vi "Init Modules.vi"(8 "error in (no error)":errorcluster, 9 "Message Queues in":T16, 11 "Settings":T1={"Support"={"Save Configuration"={"Log File Base Path"=path "", "TDMS File Reference"=refnum, "Reset"=FALSE, "Wait"=0.0, "Start Time"=0.0, "Update Rate"=1, "Channel Names"=[], "System Preset"=variant}, "LOG Configuration"={"LOG REF"=refnum, "Writer Queue"=refnum, "Log Path"=path "", "LOG"=FALSE}, "ALARM Configuration"={"LOG REF"=refnum, "Writer Queue"=refnum, "Log Path"=path "", "UPS standby"=FALSE, "status code"=5001, "SP"=[], "Over Sens Status"=[]}, "User Details"=[], "Radome Type"="", "Timer Configuration"={"Wait"=0.0, "Next Step"="", "Writer Queue"=refnum, "Reset"=FALSE, "VISA resource"="", "Status"=[], "Valve Time"=[], "Timer queue"=refnum, "Current valve"=0, "Enable"=FALSE}}, "Process"={"Test Configuration"={"current Step"=0, "Wait"=0.0, "Next Step"="", "Writer Queue"=refnum, "Reset"=FALSE, "SEQ Time"=0, "General Reset"=FALSE, "Cycles"=0, "Status"=[], "Ready"=[], "Backward"=FALSE, "Current SP"=[], "System Preset"={"Test Configuration"={"Cycles"=0, "Z Up"=0.0, "SP List"=[], "Operator"="", "Point Delay"=0, "Z Up 2"=0.0, "Cleaning In"=0.0, "Cleaning Out"=0.0, "Cleaning Cycles"=0}, "Test_Start_date"=""}, "Test Type"=enum."Calibration", "Sample Count"=0, "Local Queues"={"Cycles queue"=refnum, "Step queue"=refnum, "RES Queue"=refnum, "Clean queue"=refnum, "PS Scan queue"=refnum}, "current Clean"=0, "PS Measure Plan"=[]}}, "Report Configuration"={"Test Setting"={"Test_Num"=0, "Test_ID"=0, "Proc_ID"=0, "Max Force"=0.0, "User"="", "SN"="", "Date"=""}, "Measurements"=[], "LOG REF"=refnum, "Report Template"=path "", "Save Report path"=path "", "Data File Path"=path "", "Popup Dialog"=FALSE}, "History Data"={"Tests"=[], "Test Name"=""}, "Motor Configuration"={"Tango HW"={"VISA resource"="", "Baud Rate (115200)"=2, "lAnInterfaceType"=0, "bAShowProt"=15}, "Writer Queue"=refnum, "Status"=FALSE, "Abs Position"=[], "Axis Velocity"={"dX"=0.0, "dY"=0.0, "dZ"=0.0, "dA"=0.0}, "acceleration "=0.0, "Z direction"=enum."Up", "Position Mode"="", "plLSID"=0}, "PalmSense  Configuration"={"PalmSens.lvclass"=refnum, "Writer Queue"=refnum, "Enable"=FALSE, "Is Measuring Ref"=refnum, "Method"={"Name"="", "Method Ref"=variant}, "PS Live Curve Result"=refnum}, "Hiden Scanner Resources"={"Link"={"Connection"=enum."USB", "Host or IP address (TCP/IP)"="", "Port (Serial/USB)"="COM1"}, "VISA resource"="", "Writer Queue"=refnum, "Status"=FALSE}, "MFC Configuration"={"MFC Definition"={"MFC Port"="", "MFC Enable"=TRUE, "Baud Rate"=0, "Interface type"=enum."RS-485", "Address"=0}, "Set Point Options"={"Setpoint Value"=0.0, "Mass Flow EU 2"="", "Setpoint Source"="", "Valve Mode"=""}, "Writer Queue"=refnum, "Enable"=FALSE, "Update Rate"=0, "MRC Chamber Enable"=FALSE, "Selected Gas"="", "Address String"=""}, "Pump Configuration"={"Pump  name"=[], "Writer Queue"=refnum, "Pump Info"={"Pump Type"="", "Speed"=0, "Direction"=0, "Running"=FALSE}, "Current Pump Name"="", "Wait"=0.0, "Next Step"="", "Reset"=FALSE}} {"Pump Configuration"."Pump Info"."Direction" items=["CW", "CCW"]; "Pump Configuration"."Pump Info"."Speed" format="%03.0f"; "MFC Configuration"."Set Point Options"."Setpoint Value" min=0.0 max=0.62495 format="%.5f"; "Process"."Test Configuration"."PS Measure Plan" items=["Pretreatment settings (PS)", "Linear Sweep Voltammetry (LSV)", "Differential Pulse Voltammetry (DPV)", "Cyclic Voltammetry (CV)", "Chronoamperometry (CA)", "Chronopotentiometry (CP)", "El Imp Spectroscopy (EIS)"]; "Process"."Test Configuration"."System Preset"."Test Configuration"."SP List" format="%#.1g"; "Support"."Save Configuration"."Update Rate" min=1 max=10 step=1}) -> (0 "error out":errorcluster)   [LabVIEW 2020]
uses:
  Message Queue/All Message Queues.ctl
  Message Queue/Message Cluster.ctl
  Settings/Settings.ctl
  <instrlib>/PalmSens SDK for LabVIEW 5.10/PalmSens/PalmSens.lvclass
  Logging/Save Configuration.ctl
  LOG/LOG Configuration.ctl
  ALARM/ALARM Configuration.ctl
  Valve Control/AM Configuration.ctl
  Test Driver/Test Driver Configuration.ctl
  Test Driver/System Preset.ctl
  Test Driver/Test Type.ctl
  Report/REP Configuration.ctl
  Report/Test Setting.ctl
  MOTOR/PS Hardware Configuration.ctl
  DMM/PalmSense Hardware Configuration.ctl
  Hiden Scanner/Scanner Hardware Configuration.ctl
  MRC/MRC Configuration.ctl
  WM Pump/Pump Hardware Configuration.ctl
  REF Single  Name to ref convert.vi
  Message Queue/Enqueue Message (Single).vi
  Message Queue/Message Queue.lvlib
  Settings/Settings.lvlib
  Logging/SAVE.lvlib
  LOG/LOG.lvlib
  ALARM/QCT ALARM.lvlib
  Report/Report.lvlib
  MOTOR/MOTOR.lvlib
  Test Driver/Test Driver.lvlib
  DMM/PalmSens.lvlib
  Hiden Scanner/Hiden Scanner.lvlib
  Valve Control/Valve Control.lvlib
  MRC/MRC Module.lvlib
  WM Pump/Pump.lvlib
panel:
  in  "CMDs":string(combo)="ALARM"
  # "X"
  # "Y"
  # "Cycles"
  # "Point Delay"
  # "Up"
  # "Down"
  # "Z Axes"
  # "#C"
  # "In"
  # "Out"
  # "Cleaning [sec]"
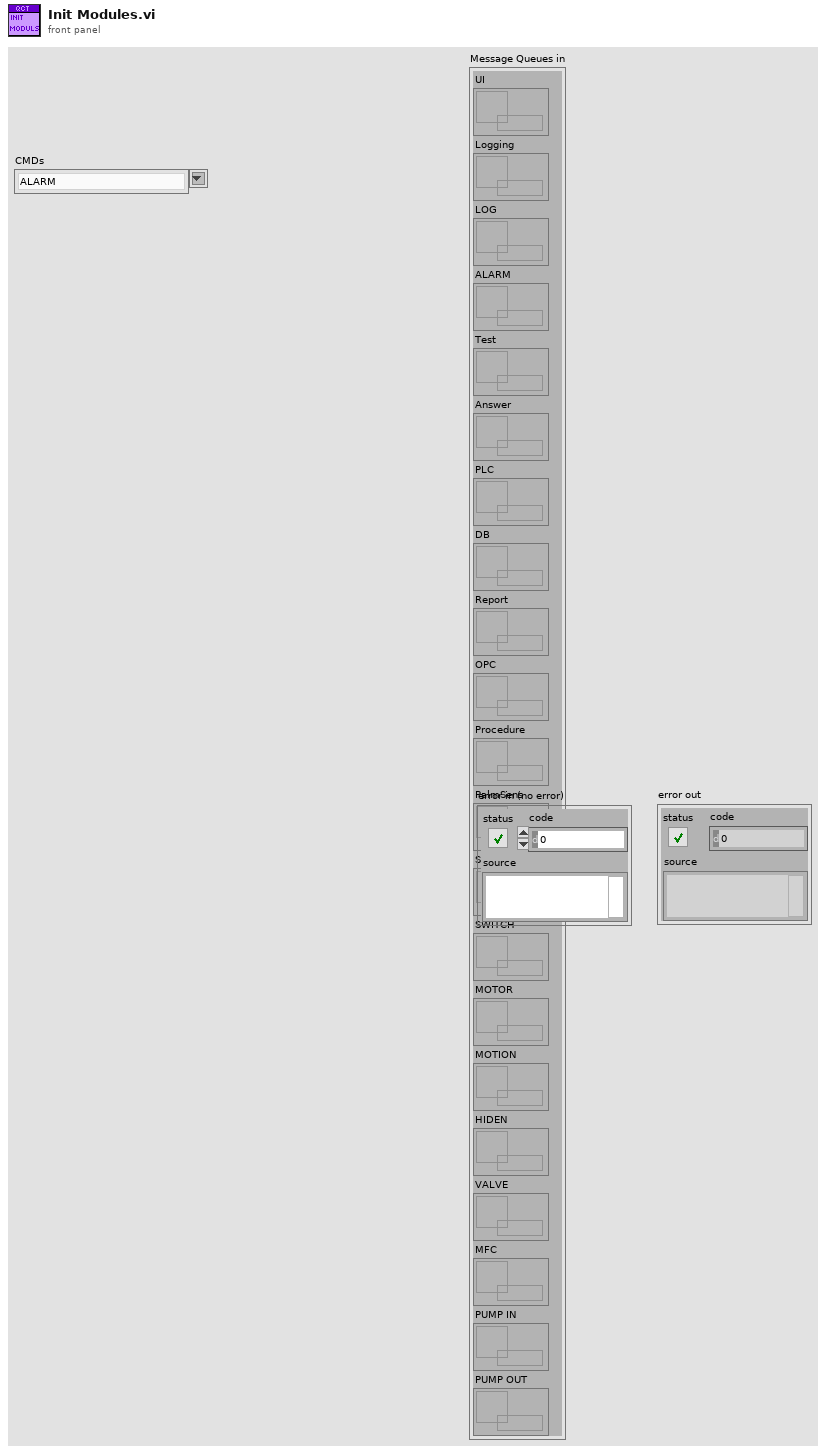
[diagram p1: front panel]
types:
  T1 = typedef "Settings.lvlib/Settings.ctl" = cluster{"Support":cluster{"Save Configuration":T2, "LOG Configuration":T3, "ALARM Configuration":T4, "User Details":string[], "Radome Type":string, "Timer Configuration":T5}, "Process":cluster{"Test Configuration":T6}, "Report Configuration":T9, "History Data":cluster{"Tests":string[][], "Test Name":string}, "Motor Configuration":T11, "PalmSense  Configuration":T12, "Hiden Scanner Resources":T13, "MFC Configuration":T14, "Pump Configuration":T15}
  T2 = typedef "SAVE.lvlib/Save Configuration.ctl" = cluster{"Log File Base Path":path, "TDMS File Reference":refnum<k34>, "Reset":bool, "Wait":dbl, "Start Time":dbl, "Update Rate":u16, "Channel Names":string[], "System Preset":variant}
  T3 = typedef "LOG.lvlib/LOG Configuration.ctl" = cluster{"LOG REF":refnum<vi>, "Writer Queue":refnum<queue>, "Log Path":path, "LOG":bool}
  T4 = typedef "QCT ALARM.lvlib/ALARM Configuration.ctl" = cluster{"LOG REF":refnum<vi>, "Writer Queue":refnum<queue>, "Log Path":path, "UPS standby":bool, "status code":i32, "SP":dbl[], "Over Sens Status":dbl[]}
  T5 = typedef "Valve Control.lvlib/AM Configuration.ctl" = cluster{"Wait":dbl, "Next Step":string, "Writer Queue":refnum<queue>, "Reset":bool, "VISA resource":refnum<visa-resource-name>, "Status":bool[], "Valve Time":dbl[], "Timer queue":refnum<queue>, "Current valve":i32, "Enable":bool}
  T6 = typedef "Test Driver.lvlib/Test Driver Configuration.ctl" = cluster{"current Step":i32, "Wait":dbl, "Next Step":string, "Writer Queue":refnum<queue>, "Reset":bool, "SEQ Time":i32, "General Reset":bool, "Cycles":i32, "Status":bool[], "Ready":bool[], "Backward":bool, "Current SP":dbl[], "System Preset":T7, "Test Type":T8, "Sample Count":i32, "Local Queues":cluster{"Cycles queue":refnum<queue>, "Step queue":refnum<queue>, "RES Queue":refnum<queue>, "Clean queue":refnum<queue>, "PS Scan queue":refnum<queue>}, "current Clean":i32, "PS Measure Plan":u16[]}
  T7 = typedef "System Preset.ctl" = cluster{"Test Configuration":cluster{"Cycles":i32, "Z Up":dbl, "SP List":dbl[][], "Operator":string, "Point Delay":i32, "Z Up 2":dbl, "Cleaning In":dbl, "Cleaning Out":dbl, "Cleaning Cycles":i32}, "Test_Start_date":string}
  T8 = typedef "Test Driver.lvlib/Test Type.ctl" = enum16{"Calibration", "Test"}
  T9 = typedef "Report.lvlib/REP Configuration.ctl" = cluster{"Test Setting":T10, "Measurements":string[][], "LOG REF":refnum<vi>, "Report Template":path, "Save Report path":path, "Data File Path":path, "Popup Dialog":bool}
  T10 = typedef "Report.lvlib/Test Setting.ctl" = cluster{"Test_Num":i32, "Test_ID":i32, "Proc_ID":i32, "Max Force":dbl, "User":string, "SN":string, "Date":string}
  T11 = typedef "MOTOR.lvlib/PS Hardware Configuration.ctl" = cluster{"Tango HW":cluster{"VISA resource":refnum<visa-resource-name>, "Baud Rate (115200)":i32, "lAnInterfaceType":i32, "bAShowProt":i32}, "Writer Queue":refnum<queue>, "Status":bool, "Abs Position":i32[], "Axis Velocity":cluster{"dX":dbl, "dY":dbl, "dZ":dbl, "dA":dbl}, "acceleration ":dbl, "Z direction":enum16{"Up", "Down"}, "Position Mode":string, "plLSID":i32}
  T12 = typedef "PalmSens.lvlib/PalmSense Hardware Configuration.ctl" = cluster{"PalmSens.lvclass":refnum<class "PalmSens.lvclass">, "Writer Queue":refnum<queue>, "Enable":bool, "Is Measuring Ref":refnum<vi>, "Method":cluster{"Name":string, "Method Ref":variant}, "PS Live Curve Result":refnum<vi>}
  T13 = typedef "Hiden Scanner.lvlib/Scanner Hardware Configuration.ctl" = cluster{"Link":cluster{"Connection":enum16{"Serial", "TCP/IP", "USB"}, "Host or IP address (TCP/IP)":string, "Port (Serial/USB)":string}, "VISA resource":refnum<visa-resource-name>, "Writer Queue":refnum<queue>, "Status":bool}
  T14 = typedef "MRC Module.lvlib/MRC Configuration.ctl" = cluster{"MFC Definition":cluster{"MFC Port":refnum<visa-resource-name>, "MFC Enable":bool, "Baud Rate":i32, "Interface type":enum32{"RS-485", "RS-232"}, "Address":i32}, "Set Point Options":cluster{"Setpoint Value":dbl, "Mass Flow EU 2":string, "Setpoint Source":string, "Valve Mode":string}, "Writer Queue":refnum<queue>, "Enable":bool, "Update Rate":u32, "MRC Chamber Enable":bool, "Selected Gas":string, "Address String":string}
  T15 = typedef "Pump.lvlib/Pump Hardware Configuration.ctl" = cluster{"Pump  name":refnum<visa-resource-name>[], "Writer Queue":refnum<queue>, "Pump Info":cluster{"Pump Type":string, "Speed":i32, "Direction":u16, "Running":bool}, "Current Pump Name":refnum<visa-resource-name>, "Wait":dbl, "Next Step":string, "Reset":bool}
  T16 = typedef "Message Queue.lvlib/All Message Queues.ctl" = cluster{"UI":refnum<queue>, "Logging":refnum<queue>, "LOG":refnum<queue>, "ALARM":refnum<queue>, "Test":refnum<queue>, "Answer":refnum<queue>, "PLC":refnum<queue>, "DB":refnum<queue>, "Report":refnum<queue>, "OPC":refnum<queue>, "Procedure":refnum<queue>, "PalmSens":refnum<queue>, "SYS 7000 Reader":refnum<queue>, "SWITCH":refnum<queue>, "MOTOR":refnum<queue>, "MOTION":refnum<queue>, "HIDEN":refnum<queue>, "VALVE":refnum<queue>, "MFC":refnum<queue>, "PUMP IN":refnum<queue>, "PUMP OUT":refnum<queue>}
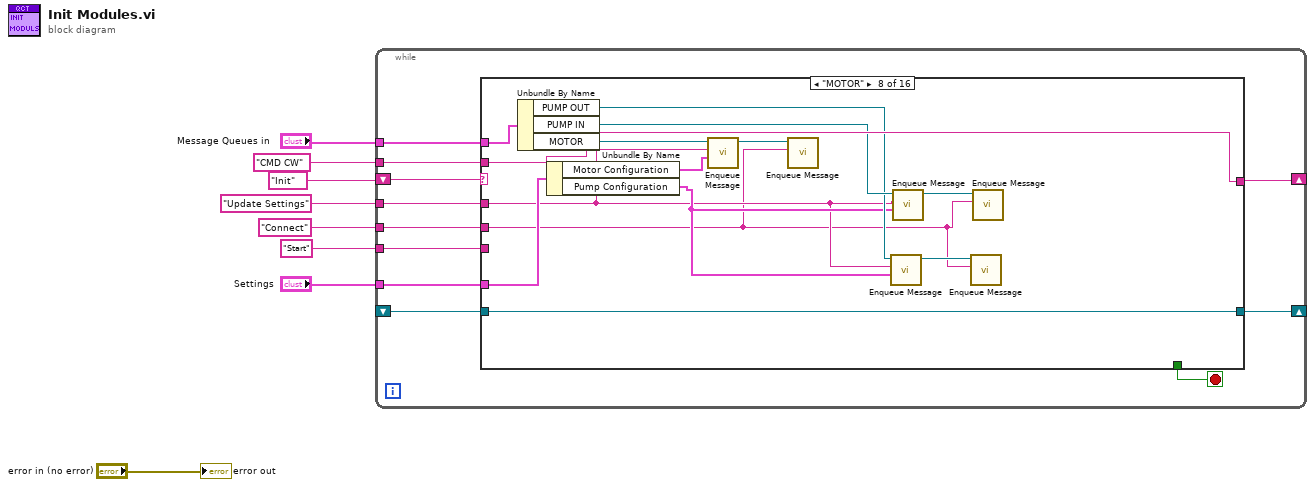
[diagram p0: block diagram]
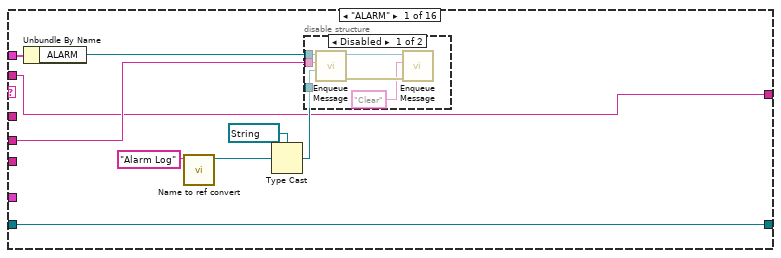
[diagram p2: hidden frame]
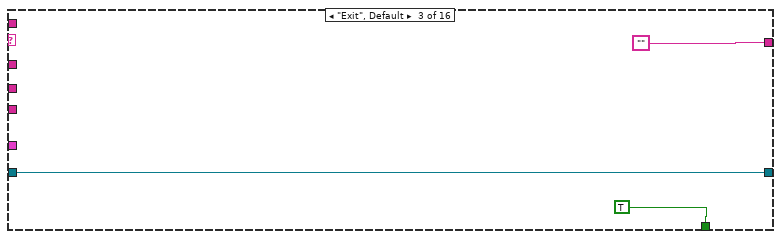
[diagram p5: hidden frame]
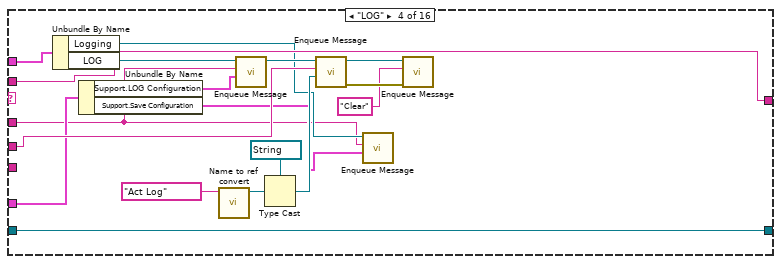
[diagram p6: hidden frame]
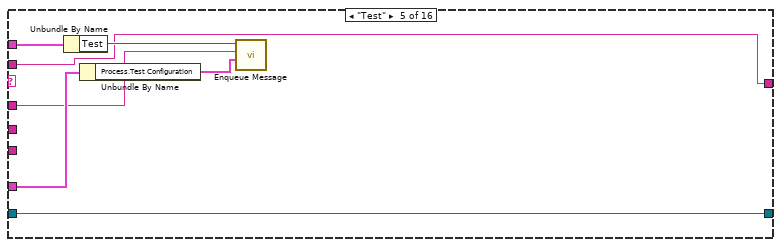
[diagram p7: hidden frame]
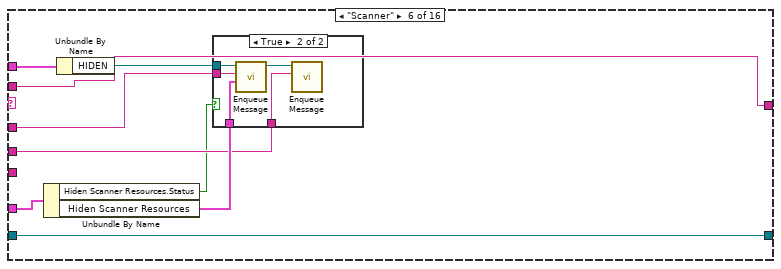
[diagram p8: hidden frame]
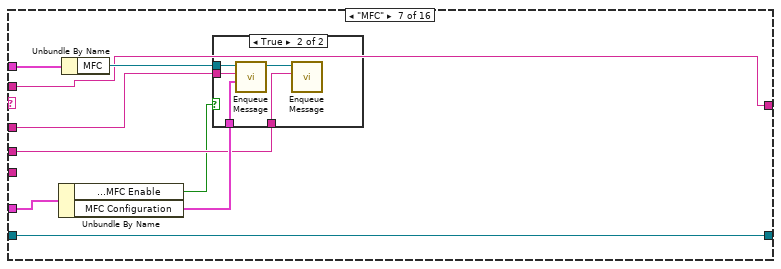
[diagram p10: hidden frame]
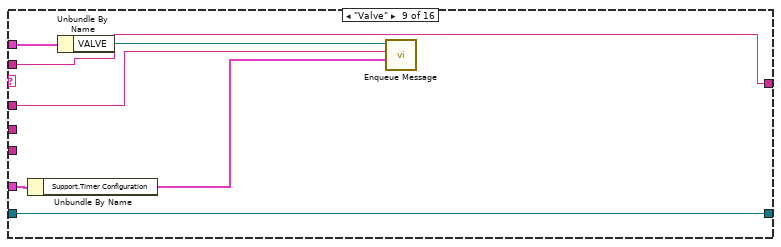
[diagram p12: hidden frame]
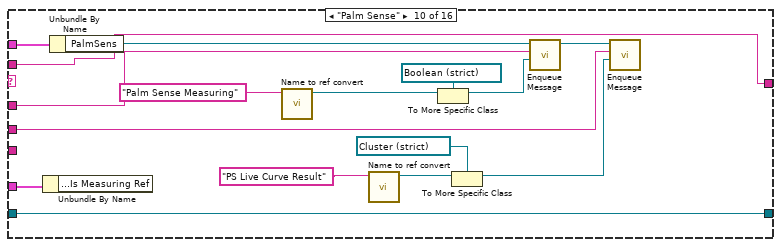
[diagram p13: hidden frame]
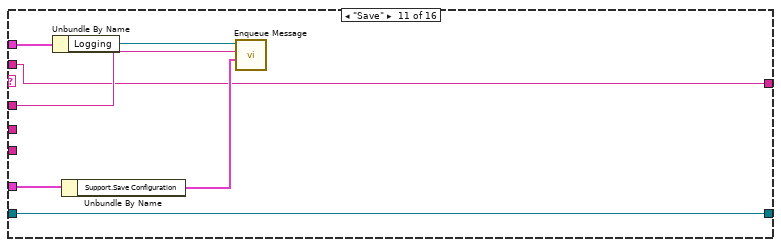
[diagram p14: hidden frame]
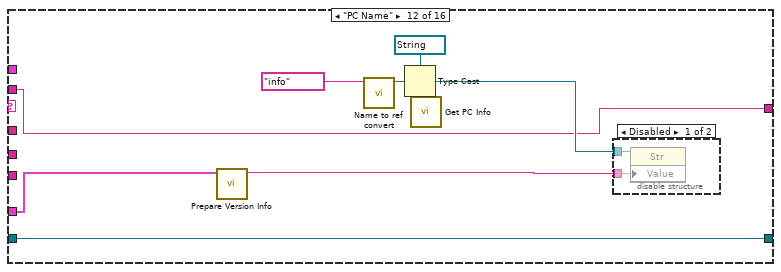
[diagram p15: hidden frame]
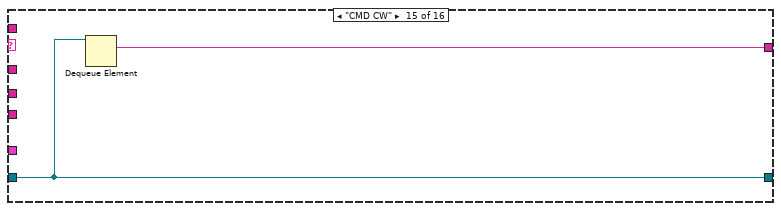
[diagram p19: hidden frame]
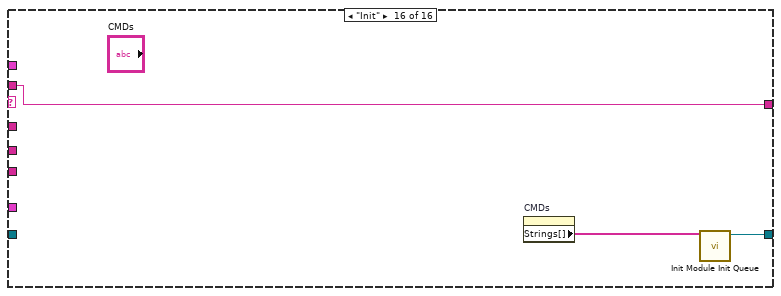
[diagram p20: hidden frame]
diagram:
  n1 = while {
    tunnel: "Message Queues in" -> [w18]
    tunnel: "Update Settings" ("Message") -> [w17]
    tunnel: "Settings" -> [w16]
    tunnel: "Connect" ("Message") -> [w15]
    shift-right: [w9] -> _
    shift-left: "Init" ("Combo Box") -> [w19]
    tunnel: "Start" ("Message") -> [w13]
    shift-right: [w11] -> _
    shift-left: _ -> [w12]
    tunnel: "CMD CW" ("Message") -> [w10]
    stop <- w14 stop-if-true
    n2 = case shown="\"MOTOR\"" w19 {
      tunnel: w18 -> [w28 _ _ w57 w64 w73 w87 w106 w113 w129 w136 _ _ _ _ _]
      tunnel: w17 -> [_ _ _ w40 w61 w70 w84 w94 w110 w125 w133 _ _ _ _ _]
      tunnel: w16 -> [_ _ _ w51 w63 w72 w86 w105 w112 w128 w135 w138 _ _ _ _]
      tunnel: w15 -> [w24 _ _ w52 _ w66 w80 w93 _ w122 _ _ _ _ _ _]
      tunnel: [w20 w35 "" w44 w58 w67 w81 w100 w107 w123 w130 w139 w147 w149 w151 w153] -> w9
      tunnel: [_ _ TRUE _ _ _ _ _ _ _ _ _ _ _ _ _] -> w14
      tunnel: w13 -> [_ _ _ _ _ _ _ _ _ _ _ _ _ _ _ _]
      tunnel: [w21 w36 w37 w45 w59 w68 w82 w101 w108 w124 w131 w140 w148 w150 w152 w154] -> w11
      tunnel: w12 -> [w21 w36 w37 w45 w59 w68 w82 w101 w108 w124 w131 w140 w148 w150 w152 _]
      tunnel: w10 -> [w20 w35 _ w44 w58 w67 w81 w100 w107 w123 w130 w139 w147 w149 _ w153]
      frame "ALARM" {
        n3 = Unbundle By Name(w28) -> ("ALARM"=w27:refnum<queue>)
        n4 = call-poly "Name to ref convert.vi"("name"="Alarm Log") -> ("First REF"=w22:refnum<vi>)  [unwired: 10 in]
        n5 = Type Cast(type=refnum<vi> refnum ("LOG"), x=w22) -> (*(type *) &x=w25:refnum<vi>)
        n6 = disable-structure shown="Disabled" {
          disable-tunnel: w27 -> [w34 _]
          disable-tunnel: w25 -> [w33 _]
          disable-tunnel: w24 -> [w29 _]
          frame Disabled {
            n7 = call-poly "Enqueue Message.vi"("Message Data"=w33, "Message"=w29, "Message Queue"=w34) -> ("error out"=w31:errorcluster, "dup Message Queue"=w32:refnum<queue>)  [unwired: 7 in]
            n8 = call-poly "Enqueue Message.vi"("error in (no error)"=w31, "Message"="Clear" ("Ready..."), "Message Queue"=w32) -> ()  [unwired: 7 in, 2 out]
          }
          frame Enabled {
          }
        }
      }
      frame "Activation" {
      }
      frame "Exit", Default {
      }
      frame "LOG" {
        n9 = Unbundle By Name(w57) -> ("Logging"=w42:refnum<queue>, "LOG"=w50:refnum<queue>)
        n10 = Unbundle By Name(w51) -> ("Support.LOG Configuration"=w48:T3, "Support.Save Configuration"=w41:T2)
        n11 = call-poly "Name to ref convert.vi"("name"="Act Log") -> ("First REF"=w46:refnum<vi>)  [unwired: 10 in]
        n12 = call-poly "Enqueue Message.vi"("Message Data"=w48, "Message"=w40, "Message Queue"=w50) -> ("dup Message Queue"=w49:refnum<queue>)  [unwired: 7 in, 1 out]
        n13 = Type Cast(type=refnum<vi> refnum ("LOG"), x=w46) -> (*(type *) &x=w55:refnum<vi>)
        n14 = call-poly "Enqueue Message.vi"("Message Data"=w55, "Message"=w52, "Message Queue"=w49) -> ("error out"=w53:errorcluster, "dup Message Queue"=w54:refnum<queue>)  [unwired: 7 in]
        n15 = call-poly "Enqueue Message.vi"("Message Data"=w41, "Message"=w40, "Message Queue"=w42) -> ()  [unwired: 7 in, 2 out]
        n16 = call-poly "Enqueue Message.vi"("error in (no error)"=w53, "Message"="Clear" ("Ready..."), "Message Queue"=w54) -> ()  [unwired: 7 in, 2 out]
      }
      frame "Test" {
        n17 = Unbundle By Name(w64) -> ("Test"=w62:refnum<queue>)
        n18 = Unbundle By Name(w63) -> ("Process.Test Configuration"=w60:T6)
        n19 = call-poly "Enqueue Message.vi"("Message Data"=w60, "Message"=w61, "Message Queue"=w62) -> ()  [unwired: 7 in, 2 out]
      }
      frame "Scanner" {
        n20 = Unbundle By Name(w72) -> ("Hiden Scanner Resources.Status"=w65:bool, "Hiden Scanner Resources"=w69:T13)
        n21 = Unbundle By Name(w73) -> ("HIDEN"=w71:refnum<queue>)
        n22 = case shown="True" w65 {
          tunnel: w71 -> [_ w78]
          tunnel: w70 -> [_ w77]
          tunnel: w69 -> [_ w76]
          tunnel: w66 -> [_ w74]
          frame False {
          }
          frame True {
            n23 = call-poly "Enqueue Message.vi"("Message Data"=w76, "Message"=w77, "Message Queue"=w78) -> ("dup Message Queue"=w75:refnum<queue>)  [unwired: 7 in, 1 out]
            n24 = call-poly "Enqueue Message.vi"("Message"=w74, "Message Queue"=w75) -> ()  [unwired: 8 in, 2 out]
          }
        }
      }
      frame "MFC" {
        n25 = Unbundle By Name(w86) -> ("MFC Configuration.MFC Definition.MFC Enable"=w79:bool, "MFC Configuration"=w83:T14)
        n26 = Unbundle By Name(w87) -> ("MFC"=w85:refnum<queue>)
        n27 = case shown="True" w79 {
          tunnel: w85 -> [_ w92]
          tunnel: w84 -> [_ w91]
          tunnel: w83 -> [_ w90]
          tunnel: w80 -> [_ w88]
          frame False {
          }
          frame True {
            n28 = call-poly "Enqueue Message.vi"("Message Data"=w90, "Message"=w91, "Message Queue"=w92) -> ("dup Message Queue"=w89:refnum<queue>)  [unwired: 7 in, 1 out]
            n29 = call-poly "Enqueue Message.vi"("Message"=w88, "Message Queue"=w89) -> ()  [unwired: 8 in, 2 out]
          }
        }
      }
      frame "MOTOR" {
        n30 = Unbundle By Name(w106) -> ("PUMP OUT"=w96:refnum<queue>, "PUMP IN"=w99:refnum<queue>, "MOTOR"=w104:refnum<queue>)
        n31 = Unbundle By Name(w105) -> ("Motor Configuration"=w102:T11, "Pump Configuration"=w95:T15)
        n32 = call-poly "Enqueue Message.vi"("Message Data"=w102, "Message"=w94, "Message Queue"=w104) -> ("dup Message Queue"=w103:refnum<queue>)  [unwired: 7 in, 1 out]
        n33 = call-poly "Enqueue Message.vi"("Message"=w93, "Message Queue"=w103) -> ()  [unwired: 8 in, 2 out]
        n34 = call-poly "Enqueue Message.vi"("Message Data"=w95, "Message"=w94, "Message Queue"=w96) -> ("dup Message Queue"=w97:refnum<queue>)  [unwired: 7 in, 1 out]
        n35 = call-poly "Enqueue Message.vi"("Message Data"=w95, "Message"=w94, "Message Queue"=w99) -> ("dup Message Queue"=w98:refnum<queue>)  [unwired: 7 in, 1 out]
        n36 = call-poly "Enqueue Message.vi"("Message"=w93, "Message Queue"=w97) -> ()  [unwired: 8 in, 2 out]
        n37 = call-poly "Enqueue Message.vi"("Message"=w93, "Message Queue"=w98) -> ()  [unwired: 8 in, 2 out]
      }
      frame "Valve" {
        n38 = Unbundle By Name(w112) -> ("Support.Timer Configuration"=w109:T5)
        n39 = Unbundle By Name(w113) -> ("VALVE"=w111:refnum<queue>)
        n40 = call-poly "Enqueue Message.vi"("Message Data"=w109, "Message"=w110, "Message Queue"=w111) -> ()  [unwired: 7 in, 2 out]
      }
      frame "Palm Sense" {
        n41 = Unbundle By Name(w128) -> ()  [unwired: 1 out]
        n42 = Unbundle By Name(w129) -> ("PalmSens"=w127:refnum<queue>)
        n43 = call-poly "Name to ref convert.vi"("name"="Palm Sense Measuring" ("Message")) -> ("First REF"=w121:refnum<vi>)  [unwired: 10 in]
        n44 = call-poly "Name to ref convert.vi"("name"="PS Live Curve Result") -> ("First REF"=w116:refnum<vi>)  [unwired: 10 in]
        n45 = To More Specific Class(target class=refnum<vi> refnum ("Palm Sense Measuring"), reference=w121) -> (specific class reference=w118:refnum<vi>)  [unwired: 1 in, 1 out]
        n46 = To More Specific Class(target class=refnum<vi> refnum ("PS Live Curve Result"), reference=w116) -> (specific class reference=w114:refnum<vi>)  [unwired: 1 in, 1 out]
        n47 = call-poly "Enqueue Message.vi"("Message Data"=w118, "Message"=w125, "Message Queue"=w127) -> ("dup Message Queue"=w126:refnum<queue>)  [unwired: 7 in, 1 out]
        n48 = call-poly "Enqueue Message.vi"("Message Data"=w114, "Message"=w122, "Message Queue"=w126) -> ()  [unwired: 7 in, 2 out]
      }
      frame "Save" {
        n49 = Unbundle By Name(w136) -> ("Logging"=w134:refnum<queue>)
        n50 = Unbundle By Name(w135) -> ("Support.Save Configuration"=w132:T2)
        n51 = call-poly "Enqueue Message.vi"("Message Data"=w132, "Message"=w133, "Message Queue"=w134) -> ()  [unwired: 7 in, 2 out]
      }
      frame "PC Name" {
        n52 = call "Prepare Version Info.vi"("Settings"=w138) -> ("String"=w137:string)  [unwired: 7 in, 3 out]
        n53 = call-poly "Name to ref convert.vi"("name"="info") -> ("First REF"=w141:refnum<vi>)  [unwired: 10 in]
        n54 = Type Cast(type=refnum<vi> refnum ("LOG"), x=w141) -> (*(type *) &x=w143:refnum<vi>)
        n55 = call "Get PC Info.vi"() -> ()  [unwired: 9 in, 3 out]
        n56 = disable-structure shown="Disabled" {
          disable-tunnel: w143 -> [w146 _]
          disable-tunnel: w137 -> [w145 _]
          frame Disabled {
            n57 = property class="Str"(reference=w146, "Value"=w145) -> ()  [unwired: 1 in, 2 out]
          }
          frame Enabled {
          }
        }
      }
      frame "SW Revision" {
      }
      frame "DB" {
      }
      frame "CMD CW" {
        n58 = Dequeue Element(queue=w152) -> (element=w151:string)  [unwired: 2 in, 3 out]
      }
      frame "Init" {
        n59 = property on="CMDs" class="CmbBox"() -> ("Strings[]"=w155:string[])  [unwired: 2 in, 2 out]
        n60 = call "Init Module Init Queue.vi"("Strings[]"=w155) -> ("Queue out"=w154:refnum<queue>)  [unwired: 10 in]
      }
    }
  }
  "error out" <- "error in (no error)"
